vi "verify acquisition finished.vi"(8 "error in (no error)":errorcluster, 11 "Save Image in":refnum<class "Save SPARC4 image.lvclass">) -> (0 "error out":errorcluster, 2 "acq finished":T1, 3 "Save Image out":refnum<class "Save SPARC4 image.lvclass">)   [LabVIEW 2018, in "Save SPARC4 image.lvclass"]
uses:
  Save SPARC4 image.lvclass
  SPARC4_Channel/SPARC4_Channel.lvclass
  Sim_CCD/Sim_CCD.lvclass
  Save Image/Save Image.lvclass
  Channel/Channel.lvclass
  C:/Users/Denis/Desktop/S4ACS/S4ACS/Channel/Channel.lvclass
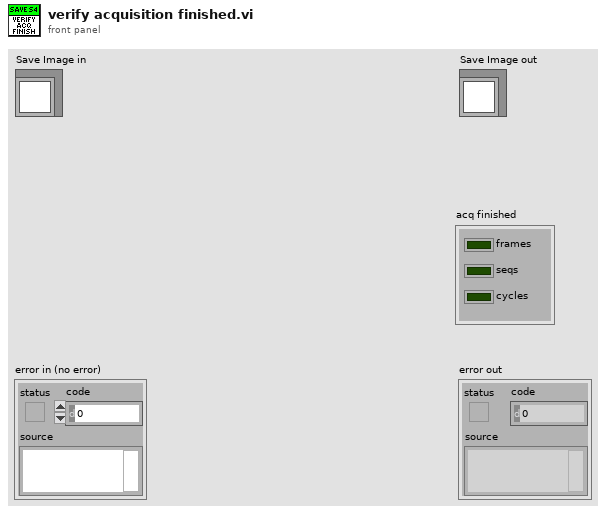
[diagram p1: front panel]
types:
  T1 = cluster{"frames":bool, "seqs":bool, "cycles":bool}
  T2 = cluster{"#SEQS":u32, "WAVEPLATE_POS":i32, "Waveplate positions":u8[]}
  T3 = cluster{"CYCLES_DONE":u16, "LAST_IMAGE_NAME":string, "USED_DISK_SPACE":u16, "IMAGE_INDEX":u32, "acquisition error":bool}
  T4 = cluster{"SEQS_DONE":u16, "S4ICS comm attempts":u8}
  T5 = cluster{"State Machine.lvclass":refnum<class "State Machine.lvclass">, "RxTx.lvclass":refnum<class "RxTx.lvclass">, "Save_Header_RxTx.lvclass":refnum<class "RxTx.lvclass">, "Status SM.lvclass":refnum<class "State Machine.lvclass">, "Status RxTx.lvclass":refnum<class "RxTx.lvclass">, "servers array":refnum<class "Server.lvclass">[], "Events log file.lvclass":refnum<class "Log File.lvclass">, "Errors log file.lvclass":refnum<class "Log File.lvclass">, "Keywords log file.lvclass":refnum<class "Log File.lvclass">, "Sim_CCD.lvclass":refnum<class "Sim_CCD.lvclass">}
  T6 = cluster{"EXPTIME":dbl, "#FRAMES":u32, "COOLER_POWER_STATUS":u16, "TEMP":i32}
  T7 = cluster{"FRAMES_DONE":u16, "CCD_STATUS":string, "CURRENT_TEMPERATURE":i16, "TEMPERATURE_STATUS":string, "FRAME_EXPOSURE_TIME":dbl, "SERIAL_NUMBER":u16, "ACQUIRING":bool, "POWER":bool, "ACS MODE":bool}
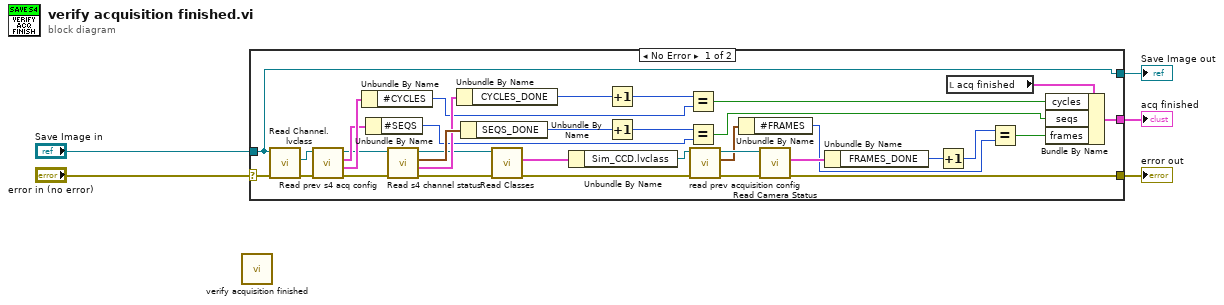
[diagram p0: block diagram]
diagram:
  n1 = call-parent "verify acquisition finished.vi"() -> ()  [unwired: 1 in]
  n2 = case shown="No Error" "error in (no error)" {
    selector: "error in (no error)" -> [w22 w41]
    tunnel: [w14 w41] -> w4
    tunnel: [w13 w40] -> w2
    tunnel: "Save Image in" -> [w13 w40]
    tunnel: [w12 _] -> w1
    frame No Error {
      n3 = call-dynamic "Read Channel.lvclass.vi"("error in (no error)"=w22, "Save Image in"=w13) -> ("error out"=w18:errorcluster, "Channel.lvclass"=w17:refnum<class "Channel.lvclass">)  [unwired: 7 in, 1 out]
      n4 = call "Read prev s4 acq config.vi"("error in (no error)"=w18, "SPARC4_Channel in"=w17) -> ("error out"=w15:errorcluster, "prev acq config"=w21:cluster{"suffix":string, "#CYCLES":u32}, "prev s4 acq config"=w20:T2, "SPARC4_Channel out"=w16:refnum<class "SPARC4_Channel.lvclass">)  [unwired: 6 in]
      n5 = Unbundle By Name(w21) -> ("#CYCLES"=w28:u32)
      n6 = Unbundle By Name(w20) -> ("#SEQS"=w19:u32)
      n7 = call "Read s4 channel status.vi"("error in (no error)"=w15, "SPARC4_Channel in"=w16) -> ("error out"=w36:errorcluster, "channel status"=w38:T3, "s4 channel status"=w39:T4, "SPARC4_Channel out"=w37:refnum<class "SPARC4_Channel.lvclass">)  [unwired: 6 in]
      n8 = Unbundle By Name(w38) -> ("CYCLES_DONE"=w11:u16)
      n9 = Unbundle By Name(w39) -> ("SEQS_DONE"=w9:u16)
      n10 = call-dynamic "Read Classes.vi"("error in (no error)"=w36, "Channel in"=w37) -> ("error out"=w31:errorcluster, "Classes"=w35:T5)  [unwired: 7 in, 1 out]
      n11 = Unbundle By Name(w35) -> ("Sim_CCD.lvclass"=w33:refnum<class "Sim_CCD.lvclass">)
      n12 = Increment(x=w11) -> (x+1=w10:u16)
      n13 = Increment(x=w9) -> (x+1=w8:u16)
      n14 = Equal?(x=w10, y=w28) -> (x = y?=w26:bool)
      n15 = Equal?(x=w8, y=w19) -> (x = y?=w25:bool)
      n16 = call "read prev acquisition config.vi"("error in (no error)"=w31, "Simulated_CCD_Camera in"=w33) -> ("error out"=w30:errorcluster, "prev acquisition configuration"=w29:T6, "Simulated_CCD_Camera out"=w32:refnum<class "Sim_CCD.lvclass">)  [unwired: 7 in]
      n17 = Unbundle By Name(w29) -> ("#FRAMES"=w23:u32)
      n18 = call "Read Camera Status.vi"("error in (no error)"=w30, "CCDCamera in"=w32) -> ("error out"=w14:errorcluster, "camera status"=w34:T7)  [unwired: 7 in, 1 out]
      n19 = Unbundle By Name(w34) -> ("FRAMES_DONE"=w7:u16)
      n20 = Increment(x=w7) -> (x+1=w6:u16)
      n21 = local read "acq finished"() -> (w27:T1)
      n22 = Equal?(x=w6, y=w23) -> (x = y?=w24:bool)
      n23 = Bundle By Name(cluster=w27, "cycles"=w26, "seqs"=w25, "frames"=w24) -> (w12:T1)
    }
    frame Error {
    }
  }
  "error out" <- w4
  "Save Image out" <- w2
  "acq finished" <- w1
